vi "Get Source List Points.vi"(8 "error in (no error)":errorcluster, 11 "VISA resource name":refnum<visa-resource-name>) -> (0 "error out":errorcluster, 1 "Source Current Points":i32, 2 "Source Voltage Points":i32, 3 "VISA resource name out":refnum<visa-resource-name>)   [LabVIEW 2018, in "Keithley 2450.lvlib"]
doc: "This command queries the length of the source list for the selected source function."
uses:
  <instrlib>/Keithley 2450/Keithley 2450.lvlib
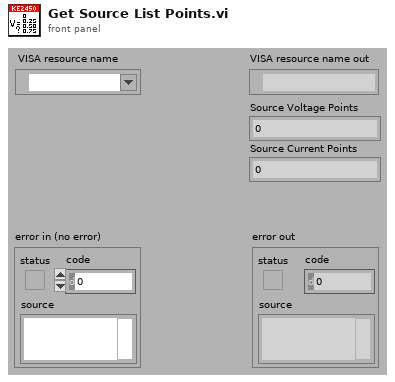
[diagram p1: front panel]
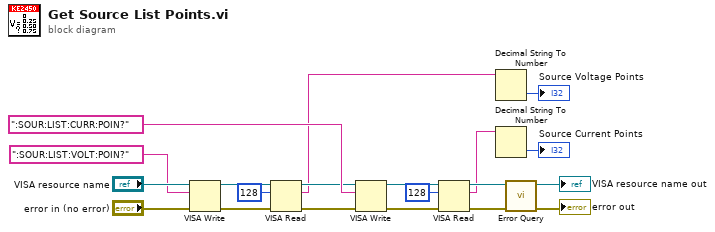
[diagram p0: block diagram]
diagram:
  n1 = VISA Write(VISA resource name="VISA resource name", write buffer=":SOUR:LIST:VOLT:POIN?", error in (no error)="error in (no error)") -> (VISA resource name out=w12:refnum<visa-resource-name>, error out=w14:errorcluster)  [unwired: 1 out]
  n2 = VISA Read(VISA resource name=w12, byte count=u32 128, error in (no error)=w14) -> (VISA resource name out=w11:refnum<visa-resource-name>, read buffer=w4:string, error out=w13:errorcluster)  [unwired: 1 out]
  n3 = VISA Write(VISA resource name=w11, write buffer=":SOUR:LIST:CURR:POIN?", error in (no error)=w13) -> (VISA resource name out=w7:refnum<visa-resource-name>, error out=w8:errorcluster)  [unwired: 1 out]
  n4 = VISA Read(VISA resource name=w7, byte count=u32 128, error in (no error)=w8) -> (VISA resource name out=w6:refnum<visa-resource-name>, read buffer=w2:string, error out=w5:errorcluster)  [unwired: 1 out]
  n5 = Decimal String To Number(string=w4) -> (number=→"Source Voltage Points":i32)  [unwired: 2 in, 1 out]
  n6 = Decimal String To Number(string=w2) -> (number=→"Source Current Points":i32)  [unwired: 2 in, 1 out]
  n7 = call <instrlib>:"Error Query.vi"("error in (no error)"=w5, "VISA resource name"=w6) -> ("error out"=→"error out":errorcluster, "VISA resource name out"=→"VISA resource name out":refnum<visa-resource-name>)  [unwired: 8 out]
